vi "Write Diagram Image.vi"(8 "error in (no error)":errorcluster, 10 "Image":T1, 11 "Data in":refnum<class "Data.lvclass">) -> (0 "error out":errorcluster, 3 "Data out":refnum<class "Data.lvclass">)   [LabVIEW 2018, in "Tracks Repair.lvlib" / "Data.lvclass"]
uses:
  Data.lvclass
  <vilib>/vision/Image Controls.llb/IMAQ Image.ctl
  Data.lvclass/Data.ctl
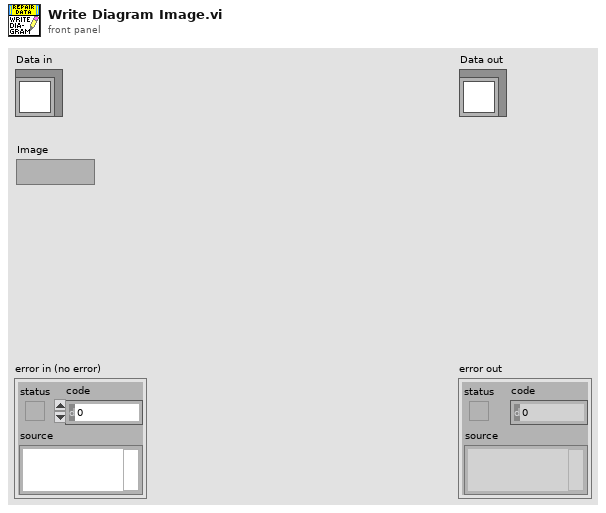
[diagram p1: front panel]
types:
  T1 = typedef "IMAQ Image.ctl" = refnum<image>
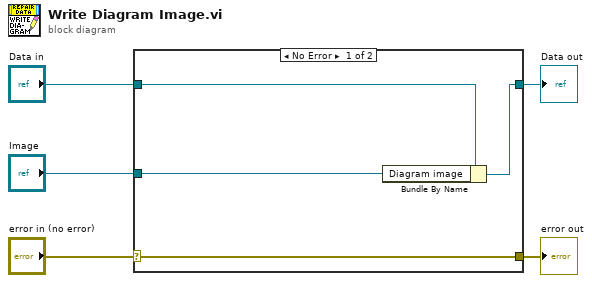
[diagram p0: block diagram]
diagram:
  n1 = case shown="No Error" "error in (no error)" {
    selector: "error in (no error)" -> [w9 w10]
    tunnel: [w9 w10] -> w4
    tunnel: [w7 w11] -> w2
    tunnel: "Data in" -> [w8 w11]
    tunnel: "Image" -> [w6 _]
    frame No Error {
      n2 = Bundle By Name(cluster=w8, "Diagram image"=w6) -> (w7:refnum<class "Data.lvclass">)
    }
    frame Error {
    }
  }
  "error out" <- w4
  "Data out" <- w2
